vi "Frac Dec Tester DSP.vi"() -> ()   [LabVIEW 2013]
uses:
  <vilib>/Platform/TimedLoop/XDataNode/timing_clust.ctl
  <vilib>/Platform/TimedLoop/XDataNode/nitl_modes.ctl
  <vilib>/Platform/TimedLoop/XDataNode/wakeup.ctl
  <instrlib>/_niInstr/DSP/v1/Shared/Public/IQ Data.ctl
  <vilib>/rvi/Emulation/niFpgaSctlEmulationGetInTimedLoop.vi
  <vilib>/rvi/Emulation/niFpgaEmulationReportErrorSimple.vi
  <vilib>/rvi/Emulation/niFpgaGetClockAttributes.vi
  <vilib>/rvi/Emulation/niFpgaCriticalErrorInLSC.vi
  <instrlib>/_niInstr/DSP/v1/FPGA/Private/Fractional Decimator/Fractional Decimator - 1 spc - 2x oc.vi
  <vilib>/rvi/FIFO/Fifo_Resource/nirvififoEmulationWriteFpgaImpl.vi
  <vilib>/rvi/DataTransferAndStorage/Container/Common/niFpgaContainerGetUniqueNameForEmu.vi
  <vilib>/rvi/eio/common/nirviEmuTemplateMethod_errors.vi
  <vilib>/rvi/FIFO/Fifo_Resource/nirvififoEmulationReadFpgaImpl.vi
  <vilib>/Platform/TimedLoop/XDataNode/XDataNode.xnode
  <vilib>/rvi/FXPMathLib/FxpInterpret/XNode/nifxpmath_Interpret.xnode
  <vilib>/rvi/DataTransferAndStorage/Container/XNode/niFpgaContainer.xnode
  <vilib>/rvi/FIFO/Fifo_Resource/nirvififoEmulationWrite.vi
  <vilib>/eio/EIONode/EIONode.xnode
  <vilib>/rvi/FIFO/Fifo_Resource/nirvififoEmulationRead.vi
  <instrlib>/_niInstr/DSP/v1/FPGA/niInstr DSP v1 FPGA.lvlib
  <vilib>/Platform/TimedLoop/XDataNode/XDNodeRunTimeDep.lvlib
  <instrlib>/_niInstr/DSP/v1/Shared/niInstr DSP v1 Shared.lvlib
panel:
  out "time outs 2":u32=3240
  out "time outs":u32=88
  in  "delay":fxp<+/-,16,0>
  in  "output sample rate":fxp<+,48,1>=0.7999944499999998 format="%#.10g"
  out "IO Module\\AI 0":i16=2980
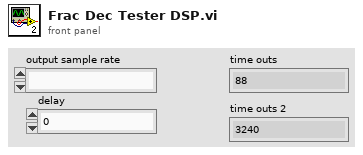
[diagram p1: front panel]
types:
  T1 = typedef "XDNodeRunTimeDep.lvlib/timing_clust.ctl" = cluster{"Expected End [f-1]":u64, "Actual End [f-1]":u64, "Finished Late? [f-1]":bool, "Expected End [i-1]":u64, "Actual End [i-1]":u64, "Finished Late? [i-1]":bool, "Expected Start [i]":u64, "Actual Start [i]":u64, "Expected Start [f]":u64, "Actual Start [f]":u64, "Source Name":string, "Structure Name":string, "Period":i64, "Deadline":i64, "Offset":i64, "Start":i64, "Priority":i32, "Timeout":i32, "Mode":T2, "Wakeup Reason":T3, "Error":errorcluster, "Source Type":string, "Secondary Source Type":string, "Global End Time":u64, "Global Start Time":u64, "Frame Duration":u64, "Iteration Duration":u64, "Assigned CPU":i32, "I/O Scan Engine Mode":u32}
  T2 = typedef "XDNodeRunTimeDep.lvlib/nitl_modes.ctl" = enum32{"No Change", "Process missed periods, maintain original phase", "Discard missed periods, maintain original phase", "Process missed periods, ignore original phase", "Discard missed periods, ignore original phase"}
  T3 = typedef "XDNodeRunTimeDep.lvlib/wakeup.ctl" = enum32{"Normal", "Aborted", "Asynchronous wakeup", "Timing source error", "Timed loop error", "Timeout"}
  T4 = typedef "niInstr DSP v1 Shared.lvlib/IQ Data.ctl" = cluster{"I":fxp<+/-,18,1>, "Q":fxp<+/-,18,1>, "overflow":bool}
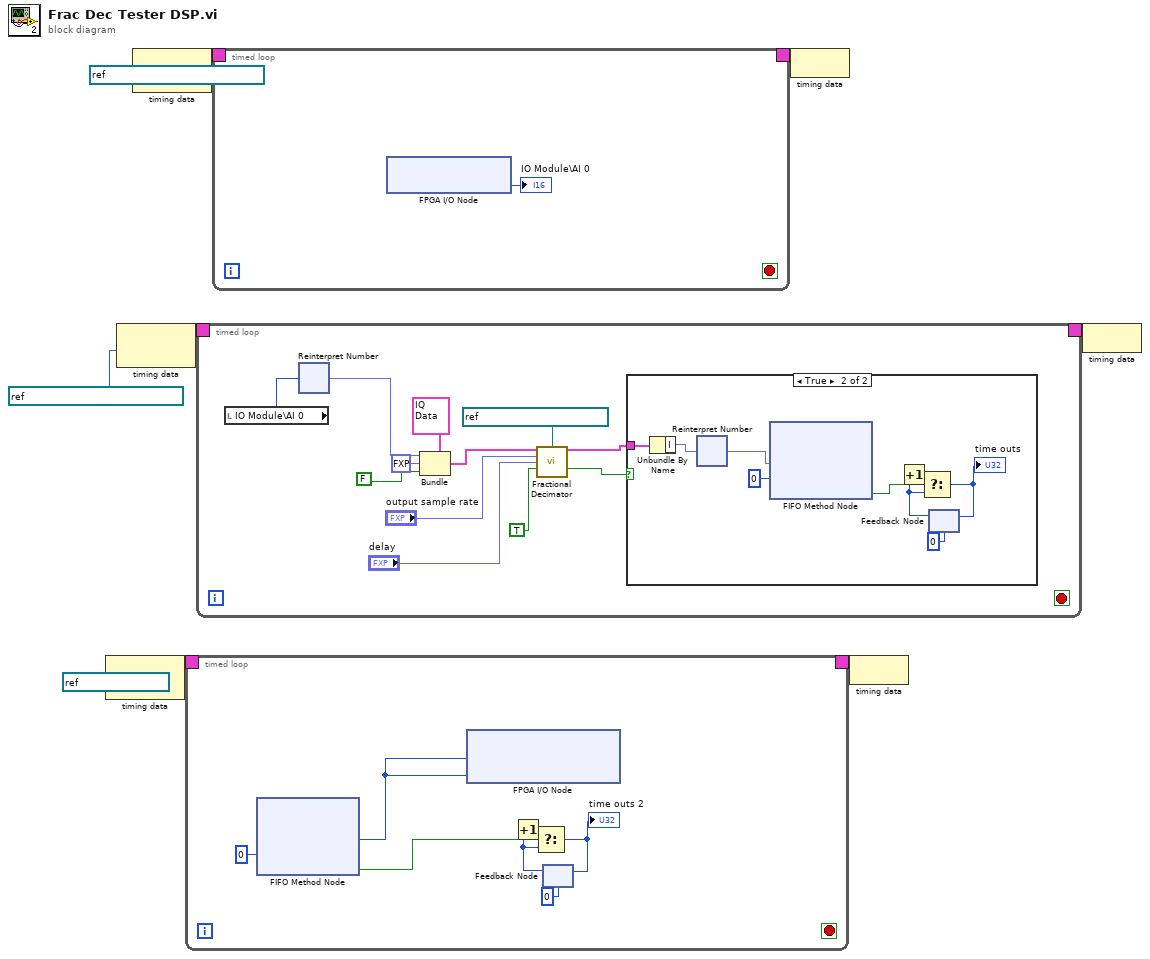
[diagram p0: block diagram]
diagram:
  n1 = node-c288(refnum<k21> "100 MHz Clock" ("Source Name")) -> (w3:T1)
  n2 = node-c288(refnum<k21> "IO Module\\Data Clock Div 2" ("Source Name")) -> (w9:T1)
  n3 = node-c288(refnum<k21> "IO Module\\Data Clock Div 2" ("Source Name")) -> (w6:T1)
  n4 = timed-loop {
    timing: w3 -> [_]
    timing-out: [_] -> w2
    stop <- _ stop-if-true
    n5 = xnode ("FIFO Method Node")("Timeout"=0) -> ("Element"=w10:i16, "Timed Out?"=w11:bool)  [unwired: 1 in, 1 out]
    n6 = xnode "FPGA I/O Node"("IO Module\\AO 0 N"=w10, "IO Module\\AO 1 N-1"=w10) -> ()  [unwired: 2 in, 2 out]
    n7 = feedback #1(u32 0) -> (w14:u32)
    n8 = Increment(x=w14) -> (x+1=w15:u32)
    n9 = Select(t=w15, s=w11, f=w14) -> (s? t:f=w13:u32)
    "time outs 2" <- w13
    n10 = feedback-in #1(w13) -> ()
  }
  n11 = timed-loop {
    timing: w9 -> [_]
    timing-out: [_] -> w8
    stop <- _ stop-if-true
    n12 = local read "IO Module\\AI 0"() -> (w21:i16)
    n13 = xnode "Reinterpret Number"("x"=w21) -> ("y"=w20:fxp<+/-,16,1>)
    n14 = Bundle(cluster=T4 {"I"=0.0, "Q"=0.0, "overflow"=FALSE} ("data in"), "I"=w20, "Q"=fxp<+/-,18,1> 0.0, "overflow"=FALSE) -> (w24:T4)
    n15 = call-poly <instrlib>:"Fractional Decimator.vi"("data in"=w24, "clock x 2"=refnum<k21> "IO Module\\Data Clock", "output sample rate"="output sample rate", "delay"="delay", "input valid"=TRUE) -> ("data out"=w26:T4, "output valid"=w23:bool)  [unwired: 8 in, 1 out]
    n16 = case shown="True" w23 {
      tunnel: w26 -> [_ w39]
      frame False {
      }
      frame True {
        n17 = Unbundle By Name(w39) -> ("I"=w32:fxp<+/-,18,1>)
        n18 = xnode "Reinterpret Number"("x"=w32) -> ("y"=w31:fxp<+/-,18,16>)
        n19 = xnode ("FIFO Method Node")("Element"=w31, "Timeout"=0) -> ("Timed Out?"=w33:bool)  [unwired: 1 in, 1 out]
        n20 = feedback #2(u32 0) -> (w35:u32)
        n21 = Increment(x=w35) -> (x+1=w34:u32)
        n22 = Select(t=w34, s=w33, f=w35) -> (s? t:f=w36:u32)
        "time outs" <- w36
        n23 = feedback-in #2(w36) -> ()
      }
    }
  }
  n24 = timed-loop {
    timing: w6 -> [_]
    timing-out: [_] -> w5
    stop <- _ stop-if-true
    n25 = xnode "FPGA I/O Node"() -> ("IO Module\\AI 0"=→"IO Module\\AI 0":i16)  [unwired: 1 in, 1 out]
  }
  n26 = node-c288(w5) -> ()
  n27 = node-c288(w2) -> ()
  n28 = node-c288(w8) -> ()
